vi "Regenerate Settings.vi"() -> (0 "Default Settings":T1)   [LabVIEW 2021, in "Settings.lvlib"]
doc: "Regenerate the default settings for the application and save to a new file.\n\nAlso copy the existing XML settings file to a .bak file."
uses:
  Settings.lvlib
  Settings.ctl
  Acquisition/Hardware Configuration.ctl
  Acquisition/Channel Settings.ctl
  Acquisition/IO Device.ctl
  Interval Timer/Repeat Interval.ctl
  Interval Timer/Interval Length.ctl
  Interval Timer/Interval Token.ctl
  Logging/Logging Configuration.ctl
  Logging/Logging Mode.ctl
  Diagnostics/Diagnostics Configuration.ctl
  Acquisition/Acquisition.lvlib
  Interval Timer/Interval Timer.lvlib
  Diagnostics/Diagnostics.lvlib
  Logging/Logging.lvlib
panel:
  out "(ignored) error out":errorcluster
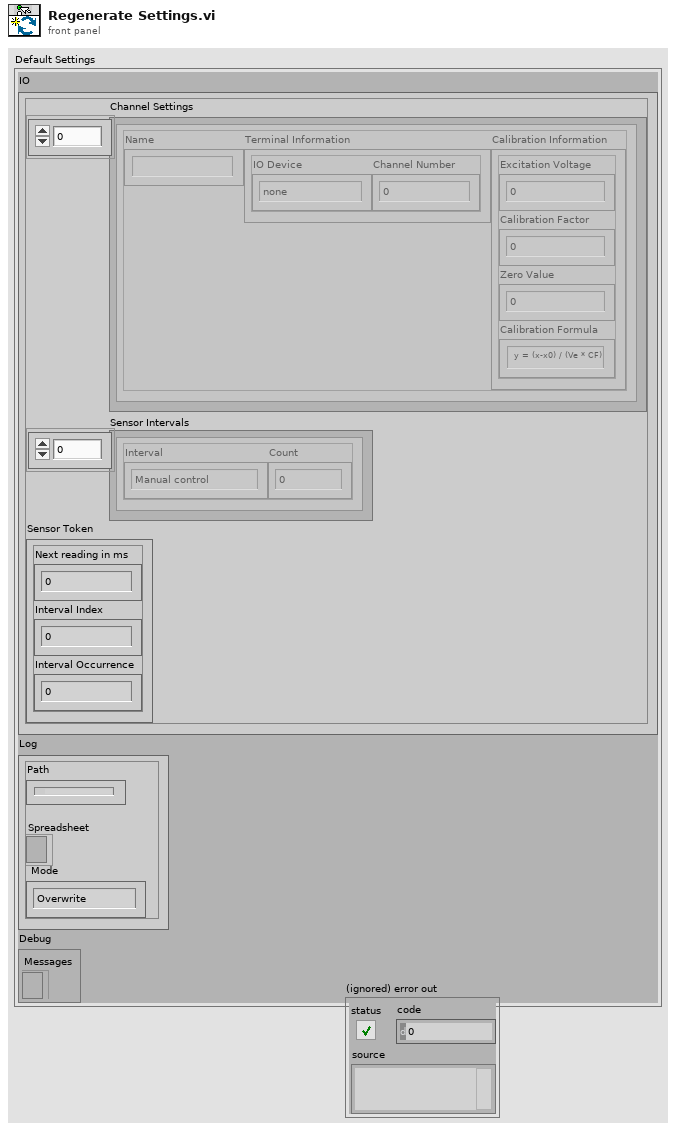
[diagram p1: front panel]
types:
  T1 = typedef "Settings.lvlib/Settings.ctl" = cluster{"IO":T2, "Log":T8, "Debug":T10}
  T2 = typedef "Acquisition.lvlib/Hardware Configuration.ctl" = cluster{"Channel Settings":T3[], "Sensor Intervals":T5[], "Sensor Token":T7}
  T3 = typedef "Acquisition.lvlib/Channel Settings.ctl" = cluster{"Name":string, "Terminal Information":cluster{"IO Device":T4, "Channel Number":i32}, "Calibration Information":cluster{"Excitation Voltage":dbl, "Calibration Factor":dbl, "Zero Value":dbl, "Calibration Formula":string}}
  T4 = typedef "Acquisition.lvlib/IO Device.ctl" = enum16{"none", "9219", "9401"}
  T5 = typedef "Interval Timer.lvlib/Repeat Interval.ctl" = cluster{"Interval":T6, "Count":i32}
  T6 = typedef "Interval Timer.lvlib/Interval Length.ctl" = enum16{"Manual control", "1 second", "10 seconds", "30 seconds", "60 seconds", "600 seconds", "1200 seconds", "3600 seconds"}
  T7 = typedef "Interval Timer.lvlib/Interval Token.ctl" = cluster{"Next reading in ms":u32, "Interval Index":i32, "Interval Occurrence":i32}
  T8 = typedef "Logging.lvlib/Logging Configuration.ctl" = cluster{"Path":path, "Spreadsheet":refnum<file>, "Mode":T9}
  T9 = typedef "Logging.lvlib/Logging Mode.ctl" = enum16{"Overwrite", "Append", "Create New"}
  T10 = typedef "Diagnostics.lvlib/Diagnostics Configuration.ctl" = cluster{"Messages":refnum<file>}
  T11 = cluster{"Excitation Voltage":dbl, "Calibration Factor":dbl, "Zero Value":dbl, "Calibration Formula":string}
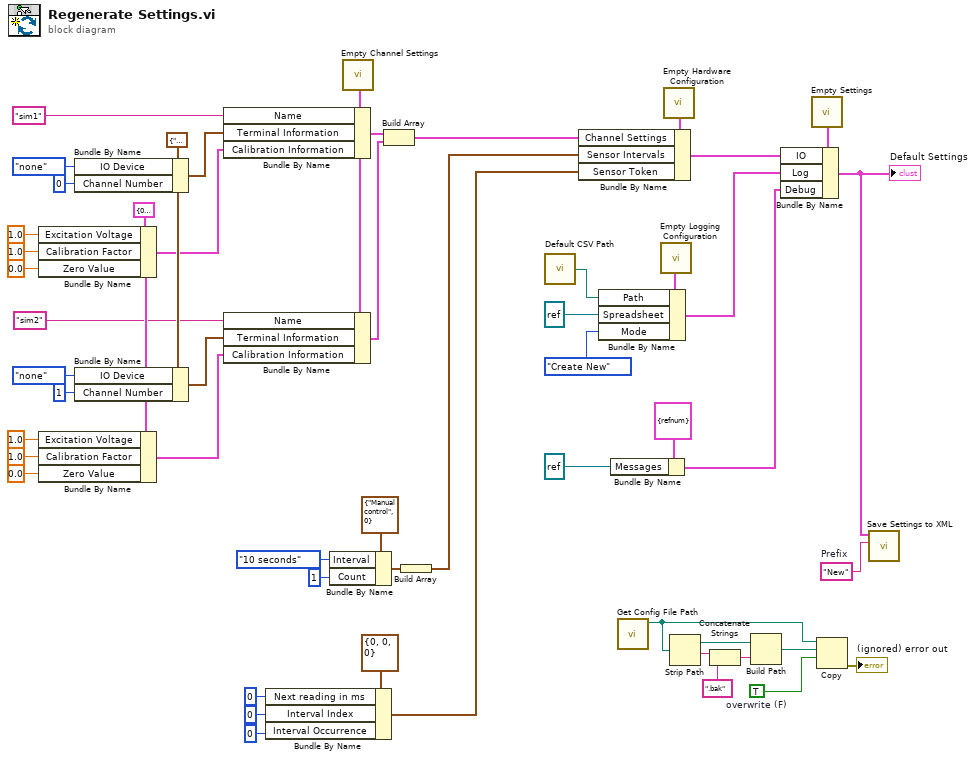
[diagram p0: block diagram]
diagram:
  w6 = TRUE  # overwrite (F)
  w27 = T11 {"Excitation Voltage"=0.0, "Calibration Factor"=0.0, "Zero Value"=0.0, "Calibration Formula"=""} ("Calibration Information")
  w29 = cluster{"IO Device":T4, "Channel Number":i32} {"IO Device"=enum."none", "Channel Number"=0} ("Terminal Information")
  w53 = "New"  # Prefix
  n1 = Bundle By Name(cluster=w27, "Excitation Voltage"=1.0, "Calibration Factor"=1.0, "Zero Value"=0.0) -> (w26:T11)
  n2 = Bundle By Name(cluster=w27, "Excitation Voltage"=1.0, "Calibration Factor"=1.0, "Zero Value"=0.0) -> (w25:T11)
  n3 = Bundle By Name(cluster=w29, "IO Device"=IO_Device."none", "Channel Number"=0) -> (w30:cluster{"IO Device":T4, "Channel Number":i32})
  n4 = Bundle By Name(cluster=w29, "IO Device"=IO_Device."none", "Channel Number"=1) -> (w28:cluster{"IO Device":T4, "Channel Number":i32})
  n5 = Bundle By Name(cluster=T7 {"Next reading in ms"=0, "Interval Index"=0, "Interval Occurrence"=0} ("Interval Token"), "Next reading in ms"=u32 0, "Interval Index"=0, "Interval Occurrence"=0) -> (w44:T7)
  n6 = Bundle By Name(cluster=T5 {"Interval"=enum."Manual control", "Count"=0} ("Repeat Interval"), "Interval"=Interval_Length."10 seconds", "Count"=1) -> (w43:T5)
  n7 = call "Empty Channel Settings.vi"() -> ("Channel Settings"=w5:T3)
  n8 = Bundle By Name(cluster=w5, "Name"="sim1", "Terminal Information"=w30, "Calibration Information"=w26) -> (w40:T3)
  n9 = Bundle By Name(cluster=w5, "Name"="sim2", "Terminal Information"=w28, "Calibration Information"=w25) -> (w31:T3)
  n10 = Build Array(w40, w31) -> (w41:T3[])
  n11 = Build Array(w43) -> (w42:T5[])
  n12 = call "Default CSV Path.vi"() -> ("CSV file path"=w39:path)
  n13 = Bundle By Name(cluster=T10 {"Messages"=refnum} ("Debug"), "Messages"=refnum<file> refnum) -> (w47:T10)
  n14 = call "Get Config File Path.vi"() -> ("XML File Path"=w8:path)  [unwired: 10 in, 1 out]
  n15 = call "Empty Logging Configuration.vi"() -> ("Logging Configuration"=w2:T8)
  n16 = Bundle By Name(cluster=w2, "Path"=w39, "Spreadsheet"=refnum<file> refnum, "Mode"=Logging_Mode."Create New") -> (w46:T8)
  n17 = call "Empty Hardware Configuration.vi"() -> ("Hardware Configuration"=w4:T2)
  n18 = Bundle By Name(cluster=w4, "Channel Settings"=w41, "Sensor Intervals"=w42, "Sensor Token"=w44) -> (w45:T2)
  n19 = Strip Path(path=w8) -> (stripped path=w12:path, name=w11:string)
  n20 = Concatenate Strings(w11, ".bak" ("string")) -> (w9:string)
  n21 = Build Path(base path=w12, name or relative path=w9) -> (appended path=w7:path)
  n22 = call "Empty Settings.vi"() -> ("Settings"=w52:T1)
  n23 = Bundle By Name(cluster=w52, "IO"=w45, "Log"=w46, "Debug"=w47) -> (w51:T1)
  "Default Settings" <- w51
  n24 = Copy(9:w6, 10:w7, 11:w8) -> (0:→"(ignored) error out":errorcluster)  [unwired: 2 in, 2 out]
  n25 = call "Save Settings to XML.vi"("Prefix"=w53, "Settings"=w51) -> ()  [unwired: 9 in, 1 out]
